vi "file pha.vi"(7 "level_of_intensity":dbl, 9 "number_of_points":i32, 10 "Path in":path, 11 "field":T1) -> (2 "Path out":string, 3 "field out":T1)   [LabVIEW 2012, in "LightPipes.lvlib"]
doc: "__declspec(dllexport) void file_pha(FIELD* field, const char* path, int number_of_points, double level_of_intensity);"
uses:
  LightPipes.lvlib
  VS Project/Debug/Lightpipes.dll
panel:
  out "error out":errorcluster
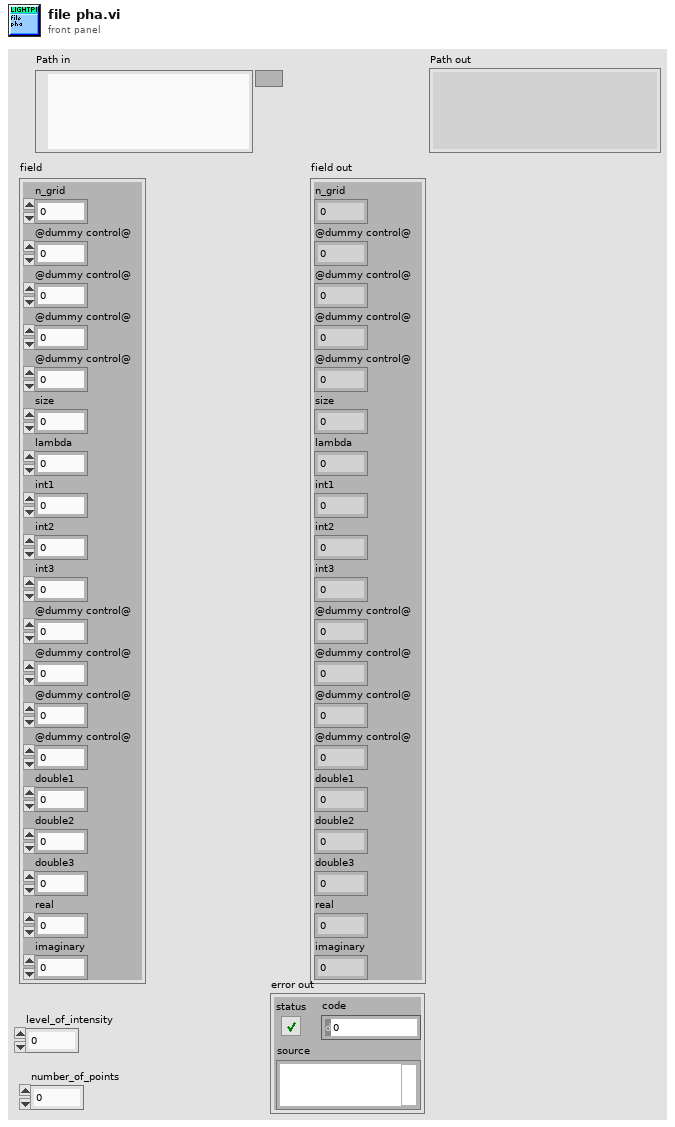
[diagram p1: front panel]
types:
  T1 = cluster{"n_grid":i32, "@dummy control@":i8, "@dummy control@":i8, "@dummy control@":i8, "@dummy control@":i8, "size":dbl, "lambda":dbl, "int1":i32, "int2":i32, "int3":i32, "@dummy control@":i8, "@dummy control@":i8, "@dummy control@":i8, "@dummy control@":i8, "double1":dbl, "double2":dbl, "double3":dbl, "real":u32, "imaginary":u32}
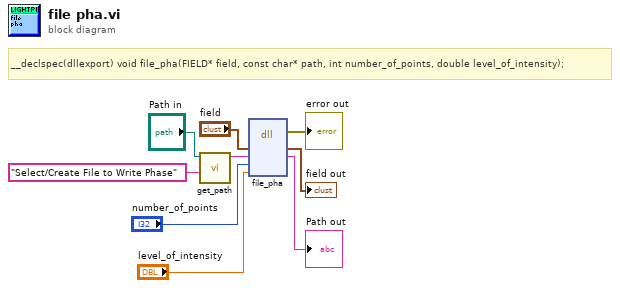
[diagram p0: block diagram]
diagram:
  # "__declspec(dllexport) void file_pha(FIELD* field, const char* path, int number_of_points, double level_of_intensity);"
  n1 = call "get_path.vi"("Message Prompt"="Select/Create File to Write Phase", "Path In"="Path in") -> ("Path out"=w4:string)  [unwired: 9 in]
  n2 = dll-call lib="C:/Users/Tri/Documents/Lightpipes/VS Project/Debug/LightPipes.*" fn="file_pha"("field"="field", "path"=w4, "number_of_points"="number_of_points", "level_of_intensity"="level_of_intensity") -> (error out=→"error out":errorcluster, "field"=→"field out":T1, "path"=→"Path out":string)  [unwired: 6 in, 1 out]
